vi "DAQNavi Create Channel(CI-Frequency).vi"(0 "task in":i32=-1, 5 "physical channels":string="DemoDevice,BID#0/cntr0", 7 "frequency measurement method":string(combo)="Omit", 9 "collection period":dbl=-1.0, 11 "error in (no error)":errorcluster) -> (4 "task out":i32, 15 "error out":errorcluster)   [LabVIEW 2020]
uses:
  DAQNavi_LV.dll
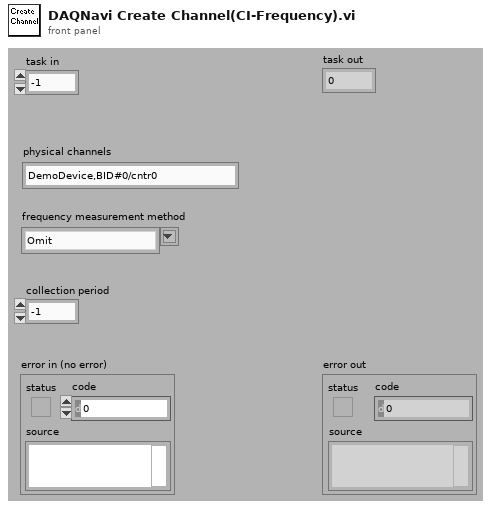
[diagram p1: front panel]
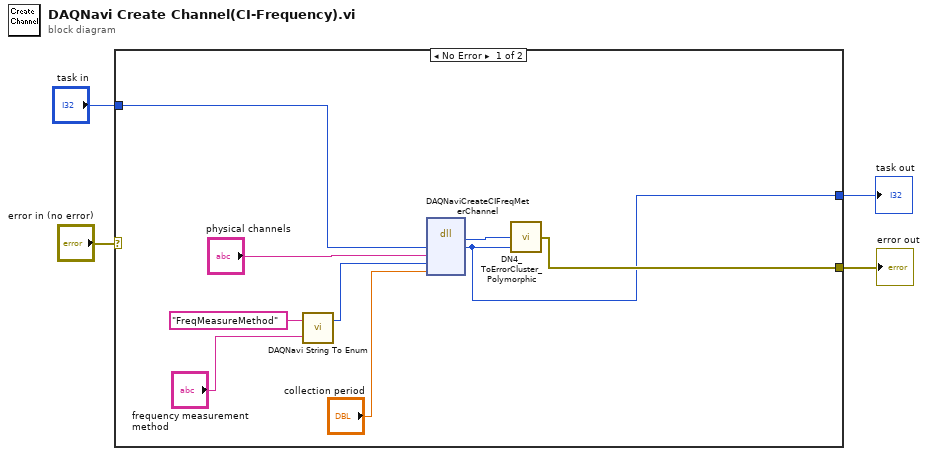
[diagram p0: block diagram]
diagram:
  n1 = case shown="No Error" "error in (no error)" {
    selector: "error in (no error)" -> [_ w14]
    tunnel: "task in" -> [w13 w15]
    tunnel: [w6 w14] -> w2
    tunnel: [w5 w15] -> w1
    frame No Error {
      n2 = call "DAQNavi String To Enum.vi"("enumString"="frequency measurement method", "enumTypeName"="FreqMeasureMethod") -> ("enumValue"=w8:i32)  [unwired: 1 out]
      n3 = dll-call lib="DAQNavi_LV.dll" fn="DAQNaviCreateCIFreqMeterChannel"("taskID"=w13, "physicalChannel"="physical channels", "method"=w8, "collectionPeriod"="collection period") -> ("return type"=w11:i32, "taskID"=w5:i32)  [unwired: 6 in, 2 out]
      n4 = call "DN4_ToErrorCluster_Polymorphic.vi"("task id"=w5, "error code"=w11) -> ("error out"=w6:errorcluster)  [unwired: 3 out]
    }
    frame Error {
    }
  }
  "error out" <- w2
  "task out" <- w1
